vi "Input Output AC Signal Test1.vi"() -> ()   [LabVIEW 2012]
uses:
  <vilib>/rvi/eio/common/nirviEmuTemplateMethod_errors.vi
  <vilib>/eio/EIONode/EIONode.xnode
panel:
  out "Output Signal 2":sgl
  in  "Sine Generator 2":sgl
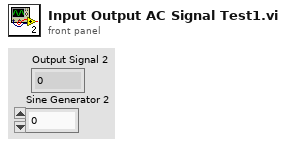
[diagram p1: front panel]
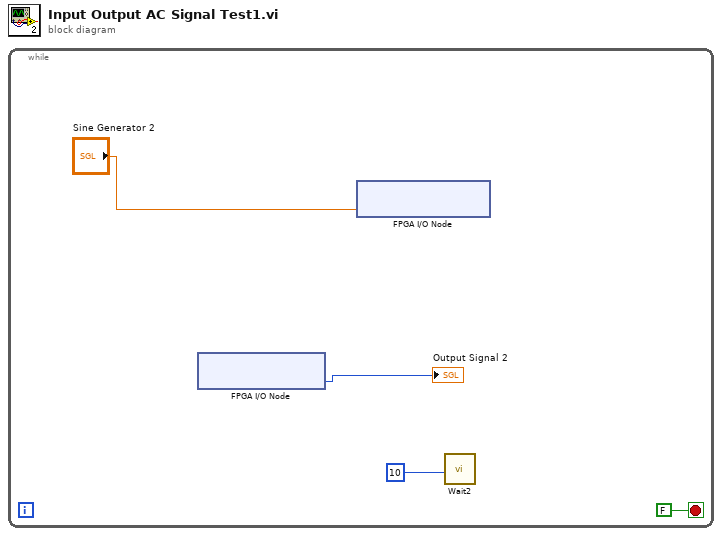
[diagram p0: block diagram]
diagram:
  n1 = while {
    stop <- FALSE stop-if-true
    n2 = xnode "FPGA I/O Node"() -> ("Connector0/AI4"=→"Output Signal 2":i16)  [unwired: 1 in, 1 out]
    n3 = xnode "FPGA I/O Node"("Connector0/AO4"="Sine Generator 2") -> ()  [unwired: 1 in, 1 out]
    n4 = call "Wait2"("Count(mSec)"=i16 10) -> ()  [unwired: 1 out]
  }
